vi "Back home.vi"   [LabVIEW 2017]
uses:
  <vilib>/myRIO/Instrument Drivers/Onboard IO/DIO/typedefs/DIO Reference.ctl
  <vilib>/myRIO/Common/Instrument Driver Framework/Utilities/typedefs/myRIO Generic Hardware Reference.ctl
  <vilib>/myRIO/Common/Instrument Driver Framework/Utilities/typedefs/Hardware Version Enum.ctl
  <vilib>/myRIO/Common/Instrument Driver Framework/Utilities/typedefs/myRIO v1.0 Reference.ctl
  <vilib>/myRIO/Common/Instrument Driver Framework/Utilities/typedefs/Generic FPGA Reference.ctl
  <vilib>/myRIO/Common/Instrument Driver Framework/myRIO v1.0/DIO/typedefs/DIO Channels List.ctl
  <vilib>/myRIO/Common/Instrument Driver Framework/myRIO v1.0/DIO/typedefs/DIO Channels Enum.ctl
  <vilib>/userdefined/High Color/nirio_resource_hc.ctl
  <vilib>/myRIO/Common/Instrument Driver Framework/Utilities/vis/Is FPGA Ref Available.vi
  <vilib>/myRIO/Common/Instrument Driver Framework/myRIO v1.0/DIO/vis/myRIO v1.1 Open DIO.vi
  <vilib>/myRIO/Instrument Drivers/Onboard IO/DIO/vis/Read.vi
  <vilib>/myRIO/Instrument Drivers/Onboard IO/DIO/vis/Write.vi
  <vilib>/myRIO/Common/Instrument Driver Framework/Utilities/vis/Validate Channels.vi
  <vilib>/myRIO/Common/Instrument Driver Framework/myRIO v1.0/DIO/vis/myRIO v1.0 Reserve DIO.vi
  <vilib>/myRIO/Common/Instrument Driver Framework/myRIO v1.0/Resource Manager/vis/myRIO v1.0 Reserve Channel List.vi
  <vilib>/myRIO/Common/Instrument Driver Framework/myRIO v1.0/DIO/vis/myRIO v1.0 Build MUX Configuration DIO.vi
  <vilib>/myRIO/Common/Instrument Driver Framework/myRIO v1.0/Resource Manager/vis/myRIO v1.0 Reserve Channel.vi
  <vilib>/myRIO/Common/Instrument Driver Framework/myRIO v1.0/Resource Manager/vis/myRIO v1.0 Unreserve Channel.vi
  <vilib>/myRIO/Common/Instrument Driver Framework/myRIO v1.0/Resource Manager/vis/myRIO v1.0 Create Configuration List.vi
  <vilib>/myRIO/Common/Instrument Driver Framework/myRIO v1.0/Resource Manager/vis/myRIO v1.0 Build Mutex Name.vi
  <vilib>/Utility/VariantDataType/GetNumericInfo.vi
  <vilib>/Utility/error.llb/Error Cluster From Error Code.vi
  <vilib>/myRIO/Common/Instrument Driver Framework/myRIO v1.0/myRIO v1.1 Open.vi
  <vilib>/myRIO/Common/Instrument Driver Framework/Utilities/vis/IO Manager.vi
  <vilib>/myRIO/Common/Instrument Driver Framework/Utilities/vis/Configuration Manager.vi
  <vilib>/myRIO/Common/Instrument Driver Framework/myRIO v1.0/Resource Manager/vis/myRIO v1.0 Configure IO.vi
  <vilib>/myRIO/Common/Instrument Driver Framework/myRIO v1.0/myRIO v1.0 Close.vi
  <vilib>/myRIO/Common/Instrument Driver Framework/myRIO v1.0/DIO/vis/myRIO v1.0 Read DIO.vi
  <vilib>/myRIO/Common/Instrument Driver Framework/myRIO v1.0/DIO/vis/myRIO v1.0 Write DIO.vi
  <vilib>/myRIO/Express VI/Onboard IO/DI/DI Express VI.xnode
  <vilib>/myRIO/Instrument Drivers/Onboard IO/DIO/vis/myRIO DIO Open.xnode
  <vilib>/myRIO/Express VI/Onboard Devices/LED/LED Express VI.xnode
  <vilib>/myRIO/Instrument Drivers/Onboard IO/DIO/DIO.lvlib
types:
  T1 = typedef "DIO.lvlib/DIO Reference.ctl" = cluster{"myRIO Reference":T2, "DIO Channels List":T6}
  T2 = typedef "myRIO Generic Hardware Reference.ctl" = cluster{"myRIO Model":T3, "myRIO Hardware Reference":T4}
  T3 = typedef "Hardware Version Enum.ctl" = enum16{"Unknown", "myRIO-1900", "myRIO-1950", "roboRIO", "NI ELVIS RIO CM"}
  T4 = typedef "myRIO v1.0 Reference.ctl" = cluster{"Generic FPGA Reference":T5, "Allow multiple opens":bool}
  T5 = typedef "Generic FPGA Reference.ctl" = refnum<k20>
  T6 = typedef "DIO Channels List.ctl" = T7[]
  T7 = typedef "DIO Channels Enum.ctl" = enum16{"Not Connected", "C/DIO0", "C/DIO1", "C/DIO2", "C/DIO3", "C/DIO4", "C/DIO5", "C/DIO6", "C/DIO7", "A/DIO0", "A/DIO1", "A/DIO2", "A/DIO3", "A/DIO4", "A/DIO5", "A/DIO6", "A/DIO7", "A/DIO8", "A/DIO9", "A/DIO10", "A/DIO11", "A/DIO12", "A/DIO13", "A/DIO14", "A/DIO15", "B/DIO0", "B/DIO1", "B/DIO2", "B/DIO3", "B/DIO4", "B/DIO5", "B/DIO6", "B/DIO7", "B/DIO8", "B/DIO9", "B/DIO10", "B/DIO11", "B/DIO12", "B/DIO13", "B/DIO14", "B/DIO15", "LED0", "LED1", "LED2", "LED3", "Button0", "DIO/DIO0", "DIO/DIO1", "DIO/DIO2", "DIO/DIO3", "DIO/DIO4", "DIO/DIO5", "DIO/DIO6", "DIO/DIO7", "DIO/DIO8", "DIO/DIO9", "SPI/CS0", "SPI/CS1", "SPI/CS2", "SPI/CS3", "LED RADIO (Green)", "LED RADIO (Red)", "LED COMM (Green)", "LED COMM (Red)", "LED MODE (Green)", "LED MODE (Red)"}
  T8 = typedef "nirio_resource_hc.ctl" = tag
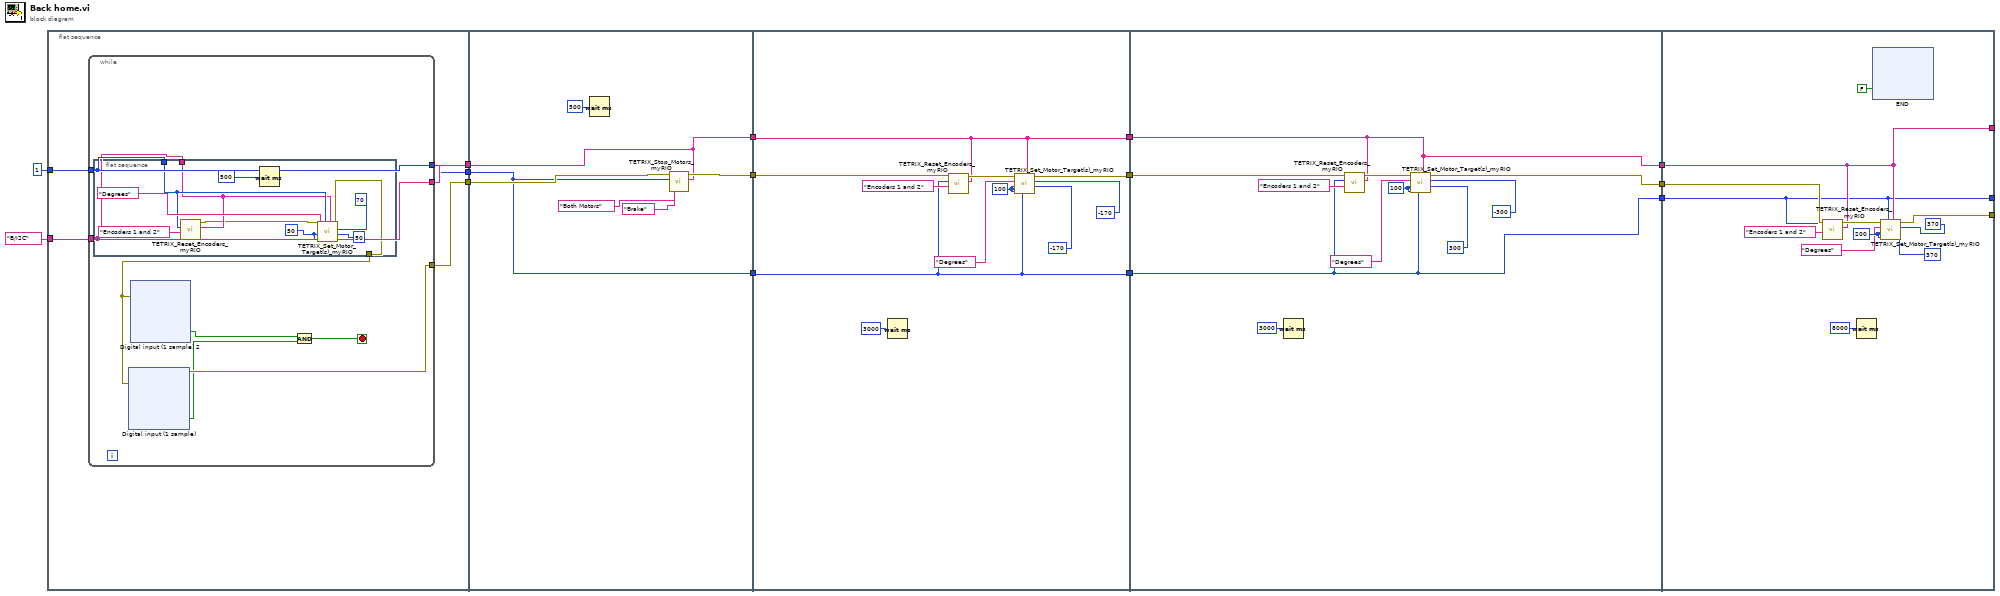
[diagram p0: block diagram]
diagram:
  n1 = flat-sequence {
    tunnel: u8 1 ("Controller ID#  (I2C Address)") -> [w19]
    tunnel: tag "B/I2C" ("myRIO MXP Port A/B") -> [w18]
    tunnel: [w17] -> w14
    tunnel: [w16] -> w13
    tunnel: [w15] -> w12
    tunnel: w14 -> [w108]
    tunnel: w13 -> [w107]
    tunnel: w12 -> [w110]
    tunnel: [w109] -> w11
    tunnel: [w108] -> w10
    tunnel: [w107] -> w9
    tunnel: w11 -> [w117]
    tunnel: [w116] -> w8
    tunnel: w10 -> [w115]
    tunnel: [w115] -> w7
    tunnel: w9 -> [w114]
    tunnel: [w114] -> w6
    tunnel: w8 -> [w128]
    tunnel: w7 -> [w127]
    tunnel: w6 -> [w125]
    tunnel: [w127] -> w5
    tunnel: [w126] -> w4
    tunnel: [w125] -> w3
    tunnel: w5 -> [w138]
    tunnel: w4 -> [w139]
    tunnel: w3 -> [w137]
    tunnel: [w138] -> _
    tunnel: [w137] -> _
    tunnel: [w136] -> _
    frame #0 {
      n2 = while {
        tunnel: w19 -> [w26]
        tunnel: w18 -> [w25]
        tunnel: [w26] -> w16
        tunnel: [w25] -> w17
        tunnel: [w24] -> w15
        stop <- w22 stop-if-true
        n3 = flat-sequence {
          tunnel: w26 -> [w66]
          tunnel: w25 -> [w65]
          tunnel: [w63] -> w23
          frame #0 {
            w71 = i16 50 ("Motor 1 Contant Speed (Degrees per Second)")
            n4 = call <vilib>:"TETRIX_Reset_Encoders_myRIO.vi"("myRIO MXP Port A/B"=w65, "Select Encoder"="Encoders 1 and 2", "Controller ID#  (I2C Address)"=w66) -> ("Error/Flow Out"=w64:errorcluster)  [unwired: 4 in]
            n5 = Wait (ms)(milliseconds to wait=u32 500) -> ()  [unwired: 1 out]
            n6 = call <vilib>:"TETRIX_Set_Motor_Target(s)_myRIO.vi"("Motor 2 Encoder Target"=50, "Motor 1 Encoder Target"=70, "myRIO MXP Port A/B"=w65, "Controller ID#  (I2C Address)"=w66, "Motor 2 Constant Speed (Degrees per Second)"=w71, "Motor 1 Contant Speed (Degrees per Second)"=w71, "Encoder Units"="Degrees", "Error/Flow In"=w64) -> ("Error/Flow Out"=w63:errorcluster)  [unwired: 1 in]
          }
        }
        n7 = xnode "Digital input (1 sample)"("error in (no error)"=w23) -> ("Right (A/DIO2 (Pin 15))"=w20:bool, "error out"=w24:errorcluster)
        n8 = xnode "Digital input (1 sample) 2"("error in (no error)"=w23) -> ("Left (A/DIO1 (Pin 13))"=w21:bool)  [unwired: 1 out]
        n9 = And(x=w21, y=w20) -> (x .and. y?=w22:bool)
      }
    }
    frame #1 {
      n10 = Wait (ms)(milliseconds to wait=u32 500) -> ()  [unwired: 1 out]
      n11 = call <vilib>:"TETRIX_Stop_Motors_myRIO.vi"("myRIO MXP Port A/B"=w108, "Stop Mode"="Brake", "Select Channel"="Both Motors", "Controller ID#  (I2C Address)"=w107, "Error/Flow In"=w110) -> ("Error/Flow Out"=w109:errorcluster)  [unwired: 2 in]
    }
    frame #2 {
      w119 = i16 100 ("Motor 1 Contant Speed (Degrees per Second)")
      n12 = Wait (ms)(milliseconds to wait=u32 3000) -> ()  [unwired: 1 out]
      n13 = call <vilib>:"TETRIX_Reset_Encoders_myRIO.vi"("myRIO MXP Port A/B"=w115, "Select Encoder"="Encoders 1 and 2", "Controller ID#  (I2C Address)"=w114, "Error/Flow In"=w117) -> ("Error/Flow Out"=w124:errorcluster)  [unwired: 3 in]
      n14 = call <vilib>:"TETRIX_Set_Motor_Target(s)_myRIO.vi"("Motor 2 Encoder Target"=-170, "Motor 1 Encoder Target"=-170, "myRIO MXP Port A/B"=w115, "Controller ID#  (I2C Address)"=w114, "Motor 2 Constant Speed (Degrees per Second)"=w119, "Motor 1 Contant Speed (Degrees per Second)"=w119, "Encoder Units"="Degrees", "Error/Flow In"=w124) -> ("Error/Flow Out"=w116:errorcluster)  [unwired: 1 in]
    }
    frame #3 {
      w134 = i16 100 ("Motor 1 Contant Speed (Degrees per Second)")
      n15 = Wait (ms)(milliseconds to wait=u32 3000) -> ()  [unwired: 1 out]
      n16 = call <vilib>:"TETRIX_Reset_Encoders_myRIO.vi"("myRIO MXP Port A/B"=w127, "Select Encoder"="Encoders 1 and 2", "Controller ID#  (I2C Address)"=w125, "Error/Flow In"=w128) -> ("Error/Flow Out"=w129:errorcluster)  [unwired: 3 in]
      n17 = call <vilib>:"TETRIX_Set_Motor_Target(s)_myRIO.vi"("Motor 2 Encoder Target"=300, "Motor 1 Encoder Target"=-300, "myRIO MXP Port A/B"=w127, "Controller ID#  (I2C Address)"=w125, "Motor 2 Constant Speed (Degrees per Second)"=w134, "Motor 1 Contant Speed (Degrees per Second)"=w134, "Encoder Units"="Degrees", "Error/Flow In"=w129) -> ("Error/Flow Out"=w126:errorcluster)  [unwired: 1 in]
    }
    frame #4 {
      w146 = i16 200 ("Motor 1 Contant Speed (Degrees per Second)")
      n18 = call <vilib>:"TETRIX_Reset_Encoders_myRIO.vi"("myRIO MXP Port A/B"=w138, "Select Encoder"="Encoders 1 and 2", "Controller ID#  (I2C Address)"=w137, "Error/Flow In"=w139) -> ("Error/Flow Out"=w142:errorcluster)  [unwired: 3 in]
      n19 = Wait (ms)(milliseconds to wait=u32 8000) -> ()  [unwired: 1 out]
      n20 = xnode "END"("LED3"=FALSE) -> ()  [unwired: 1 in, 1 out]
      n21 = call <vilib>:"TETRIX_Set_Motor_Target(s)_myRIO.vi"("Motor 2 Encoder Target"=370, "Motor 1 Encoder Target"=370, "myRIO MXP Port A/B"=w138, "Controller ID#  (I2C Address)"=w137, "Motor 2 Constant Speed (Degrees per Second)"=w146, "Motor 1 Contant Speed (Degrees per Second)"=w146, "Encoder Units"="Degrees", "Error/Flow In"=w142) -> ("Error/Flow Out"=w136:errorcluster)  [unwired: 1 in]
    }
  }
